vi "GetJoystickButton.vi"(11 "Array":bool[](array[boolean])) -> (3 "Array 2":bool[](array[boolean]))   [LabVIEW 2015]
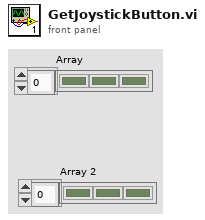
[diagram p1: front panel]
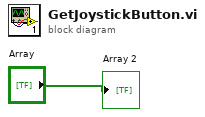
[diagram p0: block diagram]
diagram:
  "Array 2" <- "Array"
